vi "FTW-Test-Actor-Ask.vi"() -> (0 "Test Result":errorcluster)   [LabVIEW 2015]
uses:
  src/json/core/FTW-JSON-Core-Type.ctl
  src/reflection/FTW-Reflection-Types.ctl
  src/time/FTW-Time-RelativeTimer.vi
  src/socket/inbox/core/FTW-Inbox-Core-ConstructMessagePipe.vi
  src/error/FTW-ERR-PrependExplanation.vi
  src/json/FTW-JSON-Object-SetElement-String.vi
  src/json/FTW-JSON-Object-GetElement-Bool.vi
  src/json/FTW-JSON-Object-GetElement-Integer.vi
  src/json/FTW-JSON-SerializeAndDestroy.vi
  src/actor/support/FTW-Actor-DynamicLaunchOptions.vi
  src/error/FTW-ERR-Ignore.vi
  src/error/FTW-ERR-ThrowError.vi
  src/actor/request/core/FTW-Request-Core-InterpretResponse.vi
  src/socket/connector/FTW-Connector-Construct.vi
  src/error/FTW-ERR-NoErrorConstant.vi
  lib/FTW-KernelFilepath.vi
  src/json/FTW-JSON-ObjectManip-AddPair.vi
  src/socket/connector/core/FTW-Connector-Core-Ask.vi
  codegen/xnode/json/fetch/FTW-JSON-Core-GetFlattenedValue.vi
  src/error/FTW-ERR-ThrowInvalidReferenceError.vi
  src/json/core/FTW-JSON-Core-ElementType.vi
  codegen/xnode/FTW-Actor-Spawn.xnode
  src/core/type/FTW-Type-Actor-Connector.ctl
  codegen/xnode/FTW-Actor-Ask.xnode
  codegen/xnode/FTW-JSON-Fetch.xnode
  src/json/FTW-JSON-Type.ctl
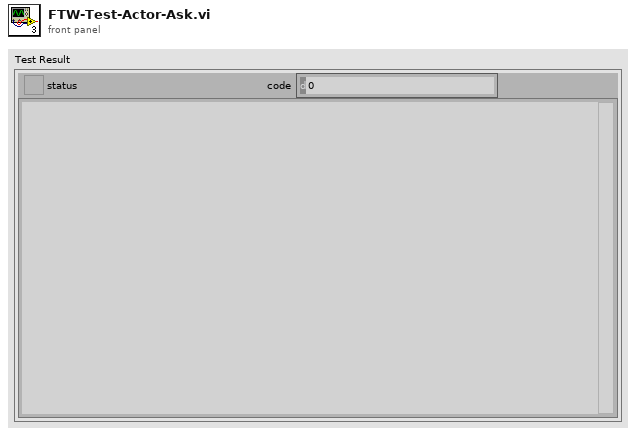
[diagram p1: front panel]
types:
  T1 = enum16{"Message is repeated verbatim", "Large message is repeated verbatim", "Fields are consumed", "Message is encoded"}[]
  T2 = typedef "FTW-Type-Actor-Connector.ctl" = refnum<data-value>
  T3 = typedef "FTW-JSON-Core-Type.ctl" = enum8{"Object", "Array", "String", "Integer", "Floating Point", "true", "false", "null", "undefined"}
  T4 = cluster{"MessageField1":string, "MessageField2":string}
  T5 = cluster{"MessageFieldToKeep":string, "MessageFieldToConsume":string}
  T6 = typedef "FTW-Type-JSON.ctl" = refnum<data-value>
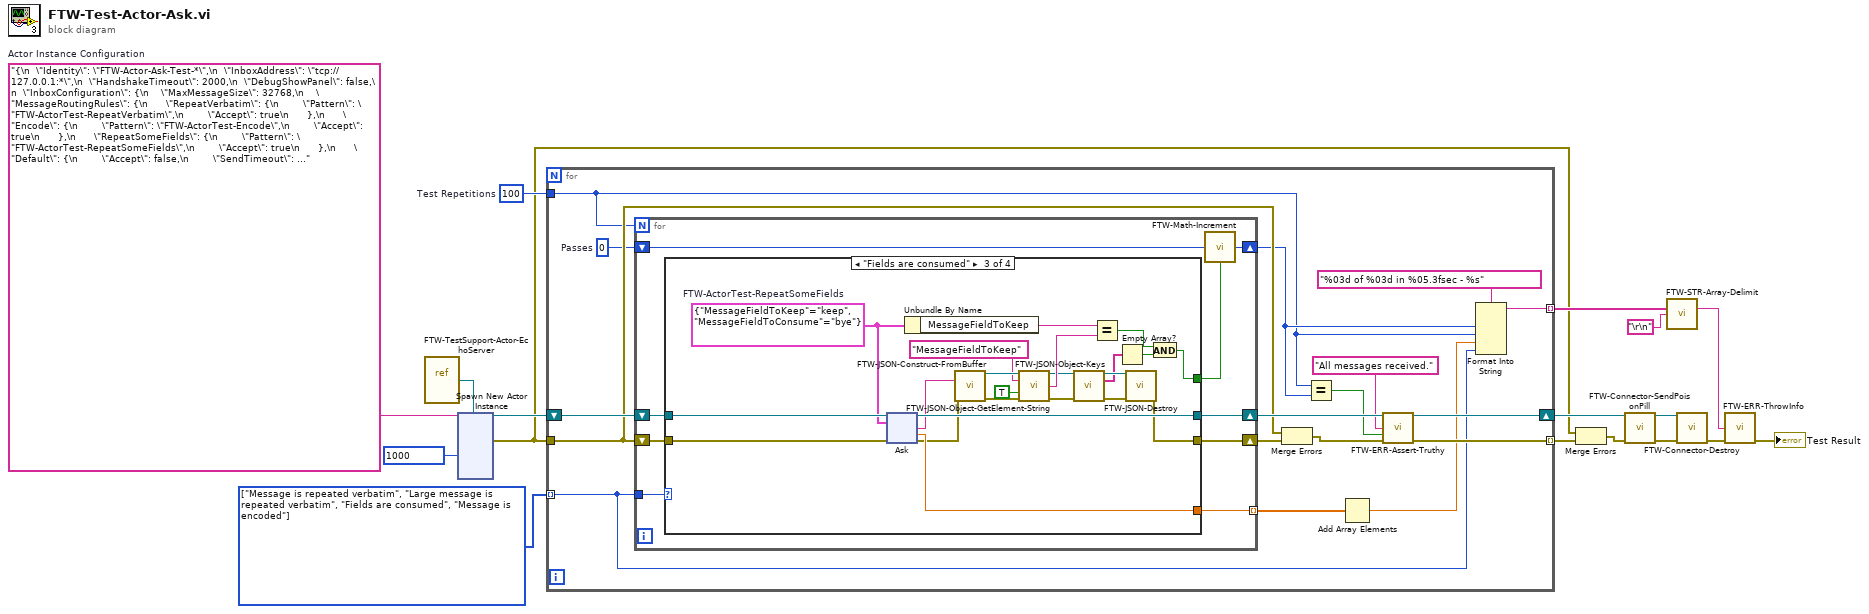
[diagram p0: block diagram]
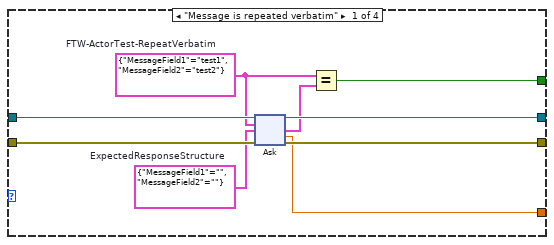
[diagram p2: hidden frame]
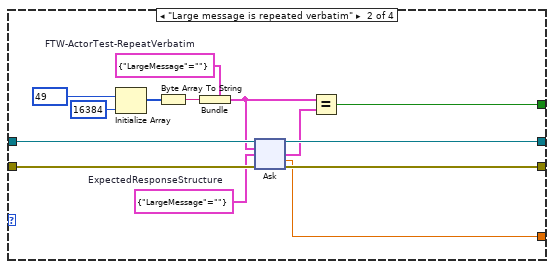
[diagram p3: hidden frame]
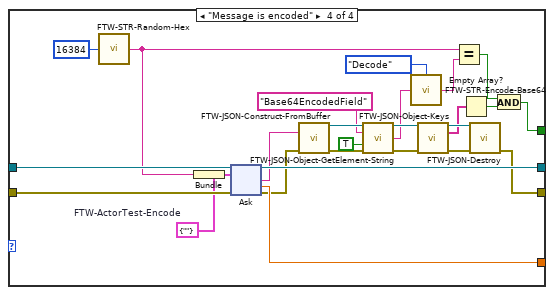
[diagram p4: hidden frame]
diagram:
  w5 = T1 [enum."Message is repeated verbatim", enum."Large message is repeated verbatim", enum."Fields are consumed", enum."Message is encoded"] items=["Message is repeated verbatim", "Large message is repeated verbatim", "Fields are consumed", "Message is encoded"]
  w7 = 100  # Test Repetitions
  w1 = "{\n  \"Identity\": \"FTW-Actor-Ask-Test-*\",\n  \"InboxAddress\": \"tcp://127.0.0.1:*\",\n  \"HandshakeTimeout\": 2000,\n  \"DebugShowPanel\": false,\n  \"InboxConfiguration\": {\n    \"MaxMessageSize\": 32768,\n    \"MessageRoutingRules\": {\n      \"RepeatVerbatim\": {\n        \"Pattern\": \"FTW-ActorTest-RepeatVerbatim\",\n        \"Accept\": true\n      },\n      \"Encode\": {\n        \"Pattern\": \"FTW-ActorTest-Encode\",\n        \"Accept\": true\n      },\n      \"RepeatSomeFields\": {\n        \"Pattern\": \"FTW-ActorTest-RepeatSomeFields\",\n        \"Accept\": true\n      },\n      \"Default\": {\n        \"Accept\": false,\n        \"SendTimeout\": 1000\n      }\n    }\n  }\n}"  # Actor Instance Configuration
  n1 = vi-ref "FTW-TestSupport-Actor-EchoServer.vi"() -> (w15:refnum<vi>)
  n2 = xnode "Spawn New Actor Instance"("Actor Instance Configuration"=w1, "Actor Instance Interface"=w15, "Idle Timeout"=1000) -> ("FTW Actor Connector"=w14:T2, "error out"=w4:errorcluster)  [unwired: 3 in, 2 out]
  n3 = for {
    shift-right: [w33] -> w16
    shift-left: w14 -> [w32]
    tunnel: [w20] -> w9 mode=indexing
    tunnel: w7 -> [w18]
    tunnel: w5 -> [w23] mode=indexing
    tunnel: w4 -> [w30]
    tunnel: [w25] -> w3 mode=indexing
    w28 = 0  # Passes
    n4 = for {
      N: w18 -> [_]
      tunnel: [w39] -> w31 mode=indexing
      shift-right: [w42] -> w33
      shift-left: w32 -> [w41]
      shift-right: [w37] -> w29
      shift-left: w30 -> [w40]
      tunnel: w23 -> [w38]
      shift-right: [w35] -> w24
      shift-left: w28 -> [w36]
      n5 = case shown="\"Fields are consumed\"" w38 {
        tunnel: [w51 w140 w237 w281] -> w42
        tunnel: w41 -> [w50 w139 w236 w280]
        tunnel: w40 -> [w49 w138 w235 w279]
        tunnel: [w46 w135 w221 w267] -> w37
        tunnel: [w47 w136 w217 w263] -> w34
        tunnel: [w45 w134 w234 w278] -> w39
        frame "Message is repeated verbatim" {
          w43 = T4 {"MessageField1"="", "MessageField2"=""}  # ExpectedResponseStructure
          w44 = T4 {"MessageField1"="test1", "MessageField2"="test2"}  # FTW-ActorTest-RepeatVerbatim
          n6 = xnode "Ask"("FTW Actor Connector"=w50, "Request"=w44, "Response Type and Defaults"=w43, "error in"=w49) -> ("FTW Actor Connector out"=w51:T2, "Response"=w48:T4, "Roundtrip Time"=w45:dbl, "error out"=w46:errorcluster)  [unwired: 1 in]
          n7 = Equal?(x=w44, y=w48) -> (x = y?=w47:bool)
        }
        frame "Large message is repeated verbatim" {
          w127 = cluster{"LargeMessage":string} {"LargeMessage"=""}  # ExpectedResponseStructure
          w133 = cluster{"LargeMessage":string} {"LargeMessage"=""}  # FTW-ActorTest-RepeatVerbatim
          n8 = Initialize Array(u8 49, 16384 ("dimension size")) -> (w129:u8[])
          n9 = Byte Array To String(unsigned byte array=w129) -> (string=w128:string)
          n10 = Bundle(cluster=w133, "LargeMessage"=w128) -> (w132:cluster{"LargeMessage":string})
          n11 = xnode "Ask"("FTW Actor Connector"=w139, "Request"=w132, "Response Type and Defaults"=w127, "error in"=w138) -> ("FTW Actor Connector out"=w140:T2, "Response"=w137:cluster{"LargeMessage":string}, "Roundtrip Time"=w134:dbl, "error out"=w135:errorcluster)  [unwired: 1 in]
          n12 = Equal?(x=w132, y=w137) -> (x = y?=w136:bool)
        }
        frame "Fields are consumed" {
          w216 = T5 {"MessageFieldToKeep"="keep", "MessageFieldToConsume"="bye"}  # FTW-ActorTest-RepeatSomeFields
          n13 = xnode "Ask"("FTW Actor Connector"=w236, "Request"=w216, "error in"=w235) -> ("FTW Actor Connector out"=w237:T2, "Response"=w232:string, "Roundtrip Time"=w234:dbl, "error out"=w222:errorcluster)  [unwired: 2 in]
          n14 = Unbundle By Name(w216) -> ("MessageFieldToKeep"=w233:string)
          n15 = call "FTW-JSON-Construct-FromBuffer.vi"("JSON String (UTF-8)"=w232, "error in"=w222) -> ("JSON"=w231:T6, "error out"=w230:errorcluster)  [unwired: 12 in]
          n16 = call "FTW-JSON-Object-GetElement-String.vi"("JSON"=w231, "Key"="MessageFieldToKeep", "Consume Value"=TRUE, "error in"=w230) -> ("JSON out"=w226:T6, "Value"=w228:string, "error out"=w225:errorcluster)  [unwired: 8 in, 1 out]
          n17 = call "FTW-JSON-Object-Keys.vi"("JSON"=w226, "error in"=w225) -> ("JSON out"=w224:T6, "Keys"=w220:string[], "error out"=w223:errorcluster)  [unwired: 11 in]
          n18 = Equal?(x=w233, y=w228) -> (x = y?=w218:bool)
          n19 = Empty Array?(array=w220) -> (empty?=w219:bool)
          n20 = call "FTW-JSON-Destroy.vi"("JSON"=w224, "error in"=w223) -> ("error out"=w221:errorcluster)  [unwired: 13 in]
          n21 = And(x=w218, y=w219) -> (x .and. y?=w217:bool)
        }
        frame "Message is encoded" {
          w261 = cluster{"MessageFieldToEncode":string} {"MessageFieldToEncode"=""}  # FTW-ActorTest-Encode
          n22 = call "FTW-STR-Random-Hex.vi"("String Length"=16384) -> ("Random Hex String"=w260:string)  [unwired: 3 in]
          n23 = Bundle(cluster=w261, "MessageFieldToEncode"=w260) -> (w256:cluster{"MessageFieldToEncode":string})
          n24 = xnode "Ask"("FTW Actor Connector"=w280, "Request"=w256, "error in"=w279) -> ("FTW Actor Connector out"=w281:T2, "Response"=w277:string, "Roundtrip Time"=w278:dbl, "error out"=w268:errorcluster)  [unwired: 2 in]
          n25 = call "FTW-JSON-Construct-FromBuffer.vi"("JSON String (UTF-8)"=w277, "error in"=w268) -> ("JSON"=w276:T6, "error out"=w275:errorcluster)  [unwired: 12 in]
          n26 = call "FTW-JSON-Object-GetElement-String.vi"("JSON"=w276, "Key"="Base64EncodedField", "Consume Value"=TRUE, "error in"=w275) -> ("JSON out"=w272:T6, "Value"=w258:string, "error out"=w271:errorcluster)  [unwired: 8 in, 1 out]
          n27 = call "FTW-STR-Encode-Base64.vi"("Input"=w258, "Direction"=enum16{"Encode", "Decode"}."Decode") -> ("Output"=w257:string)
          n28 = call "FTW-JSON-Object-Keys.vi"("JSON"=w272, "error in"=w271) -> ("JSON out"=w270:T6, "Keys"=w266:string[], "error out"=w269:errorcluster)  [unwired: 11 in]
          n29 = Equal?(x=w260, y=w257) -> (x = y?=w264:bool)
          n30 = Empty Array?(array=w266) -> (empty?=w265:bool)
          n31 = call "FTW-JSON-Destroy.vi"("JSON"=w270, "error in"=w269) -> ("error out"=w267:errorcluster)  [unwired: 13 in]
          n32 = And(x=w264, y=w265) -> (x .and. y?=w263:bool)
        }
      }
      n33 = call "FTW-Math-Increment.vi"("Initial Value"=w36, "Increment?"=w34) -> ("Final Value"=w35:i32)
    }
    n34 = Merge Errors(w30, w29) -> (w26:errorcluster)
    n35 = Equal?(x=w18, y=w24) -> (x = y?=w27:bool)
    n36 = Add Array Elements(numeric array=w31) -> (sum=w22:dbl)
    n37 = call "FTW-ERR-Assert-Truthy.vi"("Assertion"="All messages received.", "Assertion holds true?"=w27, "error in"=w26) -> ("error out"=w25:errorcluster)  [unwired: 12 in]
    n38 = Format Into String(format string="%03d of %03d in %05.3fsec - %s", w24, w18, w22, w23) -> (resulting string=w20:string)  [unwired: 2 in, 1 out]
  }
  n39 = Merge Errors(w4, w3) -> (w2:errorcluster)
  n40 = call "FTW-Connector-SendPoisonPill.vi"("Actor Connector"=w16, "error in"=w2) -> ("Actor Connector out"=w17:T2, "error out"=w6:errorcluster)  [unwired: 10 in, 2 out]
  n41 = call "FTW-STR-Array-Delimit.vi"("Array of Strings"=w9, "Delimiter"="\r\n") -> ("Delimited String"=w8:string)  [unwired: 13 in]
  n42 = call "FTW-Connector-Destroy.vi"("Actor Connector"=w17, "error in"=w6) -> ("error out"=w12:errorcluster)  [unwired: 13 in]
  n43 = call "FTW-ERR-ThrowInfo.vi"("Informational Message"=w8, "error in"=w12) -> ("error out"=→"Test Result":errorcluster)  [unwired: 13 in]
